vi "Turn.vi"(9 "number of rotations":dbl, 10 "item to rotate":refnum<class>, 11 "Rotating Tool in":refnum<class "Rotating Tool.lvclass">) -> (2 "item rotated":refnum<class>)   [LabVIEW 2023, in "Rotating Tool.lvclass"]
uses:
  Rotating Tool.lvclass
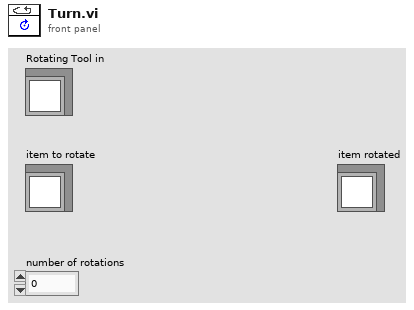
[diagram p1: front panel]
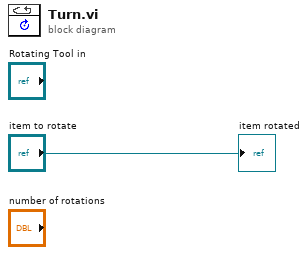
[diagram p0: block diagram]
diagram:
  "item rotated" <- "item to rotate"
